vi "cDAQ Get Digitizing Process Status.vi"(8 "error in":errorcluster, 11 "cdaq session":T1={"mclk [Hz]"=12800000.0, "ADC task"="", "mclk reference"="", "fs [Hz]"=50000.0, "queue adc cmd"=refnum, "queue adc data"=refnum, "adc proc ref"=refnum, "channels"=[], "last channels"=[], "timeout"=timestamp(0 s since 1904-01-01), "N"=1000, "mclk mode"=enum."Free running", "ext mclk source"=""} {"last channels"."Channel id" min=0 step=1; "channels"."Channel id" min=0 step=1}) -> (0 "error out":errorcluster, 1 "sweep error out":errorcluster, 3 "is running":bool)   [LabVIEW 2013]
uses:
  cDAQ Session.ctl
  low_level_old/cdaq_anal_adc_command.ctl
  low_level_old/cdaq_anal_adc_data.ctl
  cDAQ Virtual Channel.ctl
  cDAQ Master Clock Mode.ctl
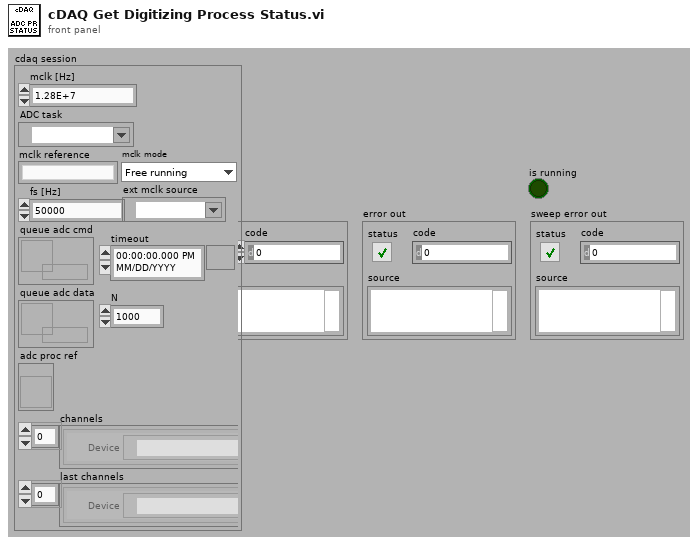
[diagram p1: front panel]
types:
  T1 = typedef "cDAQ Session.ctl" = cluster{"mclk [Hz]":dbl, "ADC task":refnum<k21>, "mclk reference":string, "fs [Hz]":dbl, "queue adc cmd":refnum<queue>, "queue adc data":refnum<queue>, "adc proc ref":refnum<vi>, "channels":T2[], "last channels":T2[], "timeout":timestamp, "N":i32, "mclk mode":T3, "ext mclk source":tag}
  T2 = typedef "cDAQ Virtual Channel.ctl" = cluster{"Device":tag, "Channel id":i32, "btn clr":bool, "btn up":bool, "btn down":bool}
  T3 = typedef "cDAQ Master Clock Mode.ctl" = enum16{"Free running", "Export master clock", "Import master clock"}
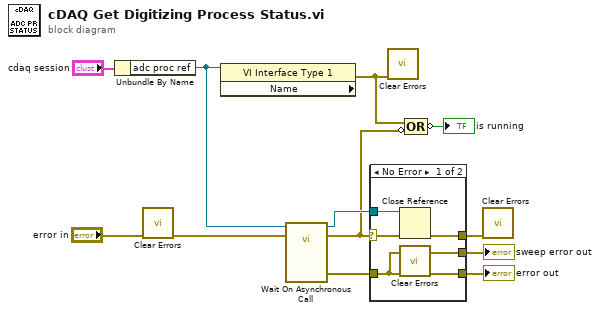
[diagram p0: block diagram]
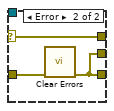
[diagram p2: hidden frame]
diagram:
  n1 = Unbundle By Name("cdaq session") -> ("adc proc ref"=w4:refnum<vi>)
  n2 = call <vilib>:"Clear Errors.vi"("error in (no error)"="error in") -> ("error out"=w7:errorcluster)  [unwired: 6 in]
  n3 = property class="VI Interface Type 1" props=["Name"](reference=w4) -> (error out=w3:errorcluster)  [unwired: 1 in, 2 out]
  n4 = call-by-ref "Wait On Asynchronous Call"(reference=w4, error in=w7) -> (reference out=w10:refnum<vi>, error out=w2:errorcluster, 0:"error out"=w8:errorcluster)  [unwired: 11 in]
  n5 = case shown="No Error" w2 {
    selector: w2 -> [w17 w20]
    tunnel: w10 -> [w16 _]
    tunnel: [w15 w20] -> w9
    tunnel: [w13 w18] -> w12
    tunnel: w8 -> [w14 w19]
    tunnel: [w14 w18] -> w11
    frame No Error {
      n6 = Close Reference(reference=w16, error in (no error)=w17) -> (error out=w15:errorcluster)
      n7 = call <vilib>:"Clear Errors.vi"("error in (no error)"=w14) -> ("error out"=w13:errorcluster)  [unwired: 6 in]
    }
    frame Error {
      n8 = call <vilib>:"Clear Errors.vi"("error in (no error)"=w19) -> ("error out"=w18:errorcluster)  [unwired: 6 in]
    }
  }
  "error out" <- w12
  "sweep error out" <- w11
  n9 = call <vilib>:"Clear Errors.vi"("error in (no error)"=w3) -> ()  [unwired: 6 in, 1 out]
  n10 = Compound Arithmetic op=OR(w3, invert w2) -> (invert →"is running":bool)
  n11 = call <vilib>:"Clear Errors.vi"("error in (no error)"=w9) -> ()  [unwired: 6 in, 1 out]
